vi "Update_footer.vi"(11 "Footer info":T1) -> (3 "File text out":string)   [LabVIEW 2017, in "labview-standard-library.lvlib" / "automode-scripting.lvlib"]
uses:
  automode-scripting.lvlib
  Footer_cluster.ctl
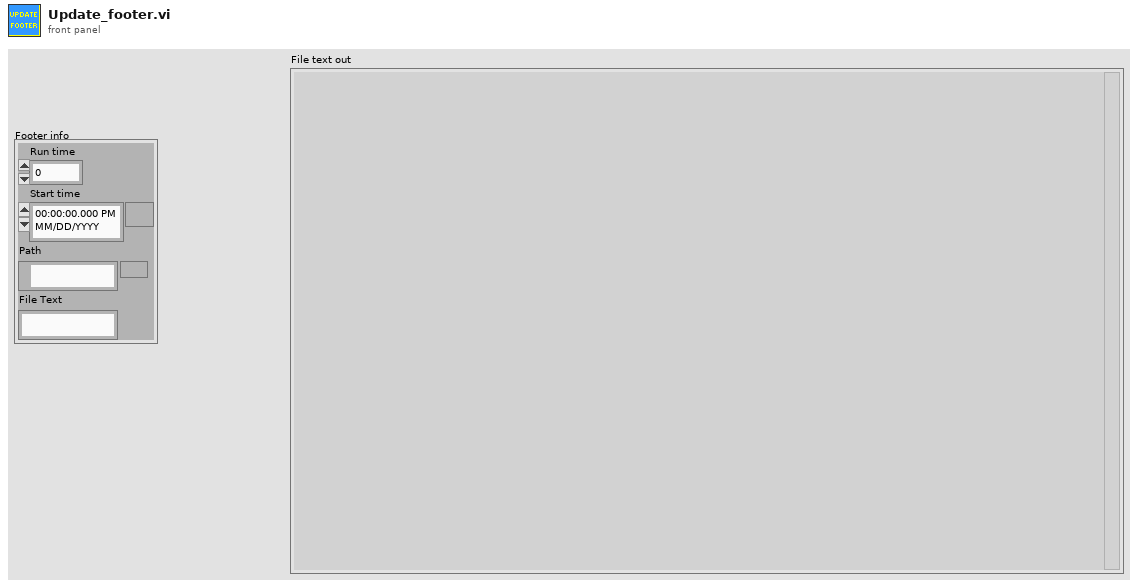
[diagram p1: front panel]
types:
  T1 = typedef "labview-standard-library.lvlib/automode-scripting.lvlib/Footer_cluster.ctl" = cluster{"Run time":dbl, "Start time":timestamp, "Path":path, "File Text":string}
  T2 = enum16{"open", "replace", "create", "open or create", "replace or create", "replace or create with confirmation"}
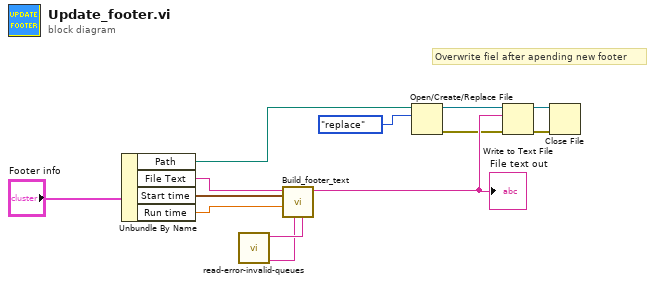
[diagram p0: block diagram]
diagram:
  # "Overwrite fiel after apending new footer"
  n1 = Unbundle By Name("Footer info") -> ("Path"=w4:path, "File Text"=w3:string, "Start time"=w11:timestamp, "Run time"=w10:dbl)
  n2 = call "read-error-invalid-queues.vi"() -> ("Subsystem error string"=w1:string, "Invalid code string"=w2:string)  [unwired: 10 in]
  n3 = call "Build_footer_text.vi"("Invalid line"=w2, "Error string"=w1, "Run time"=w10, "Start time"=w11, "File Text"=w3) -> ("file w/footer"=w13:string)  [unwired: 6 in]
  "File text out" <- w13
  n4 = Open/Create/Replace File(file path (use dialog)=w4, operation (0:open)=T2."replace") -> (refnum out=w8:refnum<file>, error out=w9:errorcluster)  [unwired: 4 in, 1 out]
  n5 = Write to Text File(file (use dialog)=w8, text=w13, error in=w9) -> (refnum out=w5:refnum<file>, error out=w6:errorcluster)  [unwired: 1 in, 1 out]
  n6 = Close File(refnum=w5, error in=w6) -> ()  [unwired: 2 out]
